vi "dfd_Bilinear Prewarping of f.vi"(1 "freq specs [Hz]":T1) -> (0 "prewarped freq specs [Hz]":T1)   [LabVIEW 2017, in "NI_DigFilter_Design.lvlib"]
uses:
  <vilib>/addons/Digital Filter Design/NI_DigFilter_Design.lvlib
  <vilib>/addons/Digital Filter Design/_Objects.llb/DFD Filter Frequence Specification (Design).ctl
  <vilib>/addons/Digital Filter Design/NI_DigFilterLicensed.lvlib
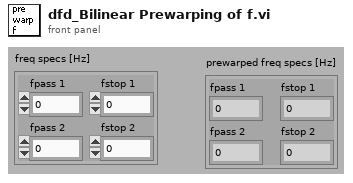
[diagram p1: front panel]
types:
  T1 = typedef "NI_DigFilterLicensed.lvlib/DFD Filter Frequence Specification (Design).ctl" = cluster{"fpass 1":dbl, "fstop 1":dbl, "fpass 2 ":dbl, "fstop 2":dbl}
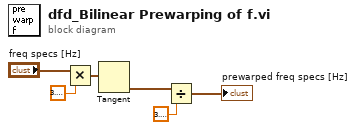
[diagram p0: block diagram]
diagram:
  n1 = Multiply(x="freq specs [Hz]", y=3.141592653589793) -> (x*y=w6:T1)
  n2 = Tangent(1:w6) -> (0:w3:T1)
  n3 = Divide(x=w3, y=3.141592653589793) -> (x/y=→"prewarped freq specs [Hz]":T1)
